vi "FEA_Model_Sample.vi"(8 "error in (no error)":errorcluster, 9 "include extremes":bool=TRUE, 10 "standard_deviation":dbl, 11 "FEA_Model in":refnum<class "FEA_Model.lvclass">) -> (0 "error out":errorcluster, 3 "FEA_Model out":refnum<class "FEA_Model.lvclass">)   [LabVIEW 2021, in "FEA_Model.lvclass"]
uses:
  FEA_Model.lvclass
  FEA_Model.lvclass/FEA_Model.ctl
  de957b9d-3b39-418b-bf55-63c688e4ea67.vi
  fbdf095a-6d06-4ca0-9642-1e4932d1de12.vi
  <vilib>/gmath/statdist.llb/Normal PDF.vi
  <vilib>/Comparison/Less/Less Functor/Less Functor.lvclass
  <vilib>/gmath/NI_Gmath.lvlib
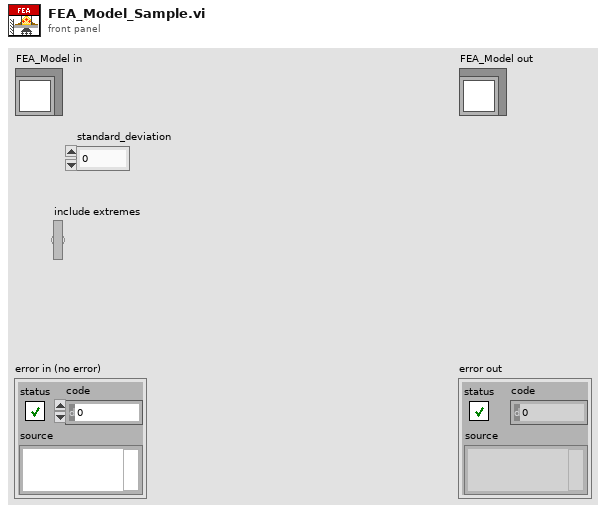
[diagram p1: front panel]
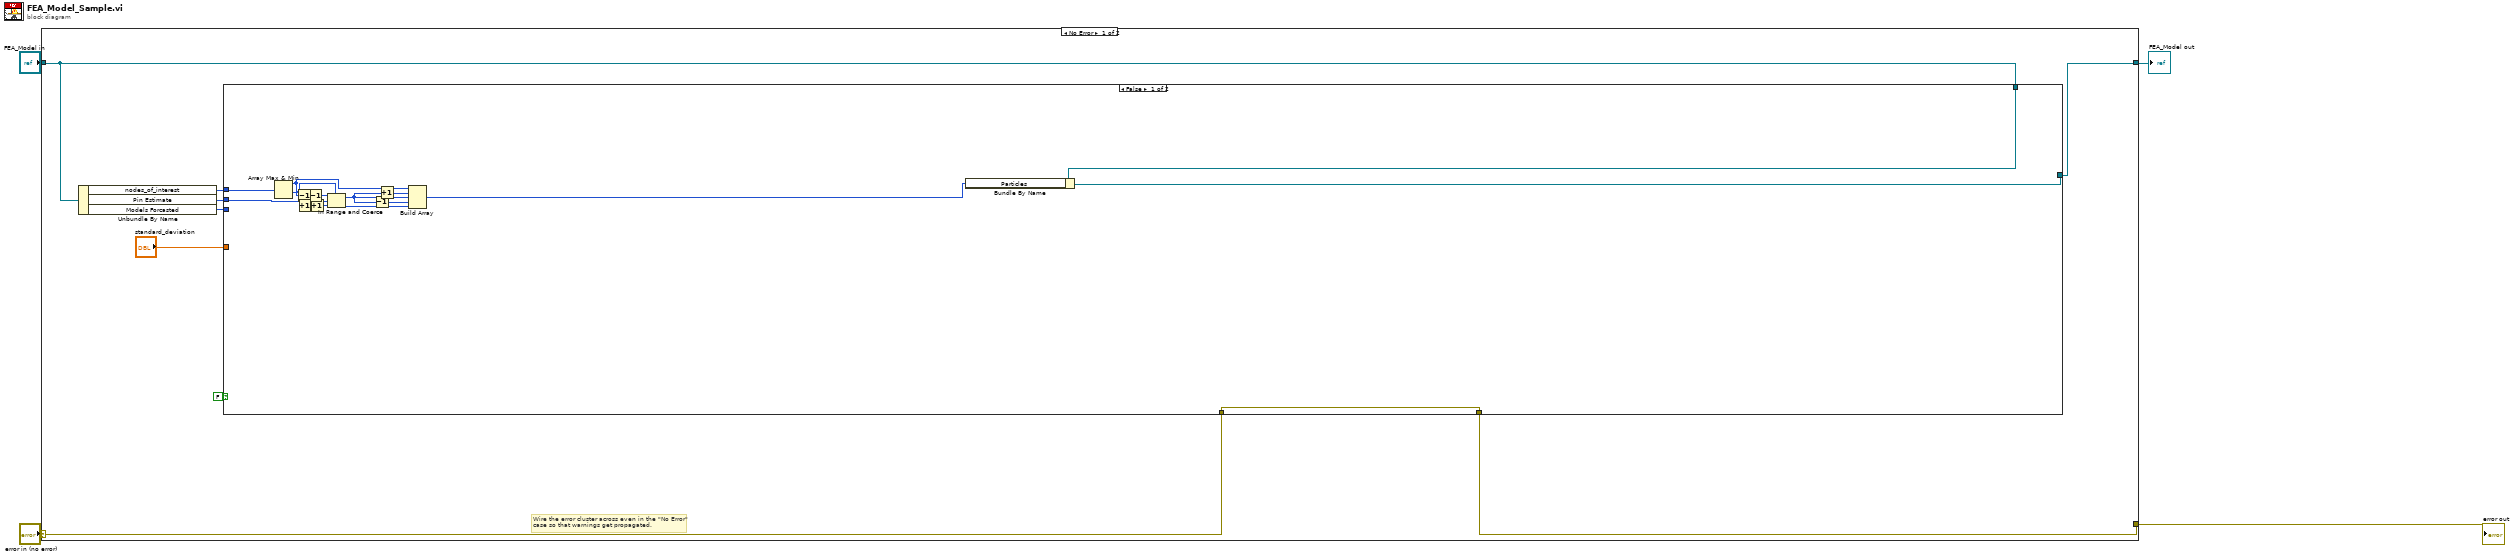
[diagram p0: block diagram]
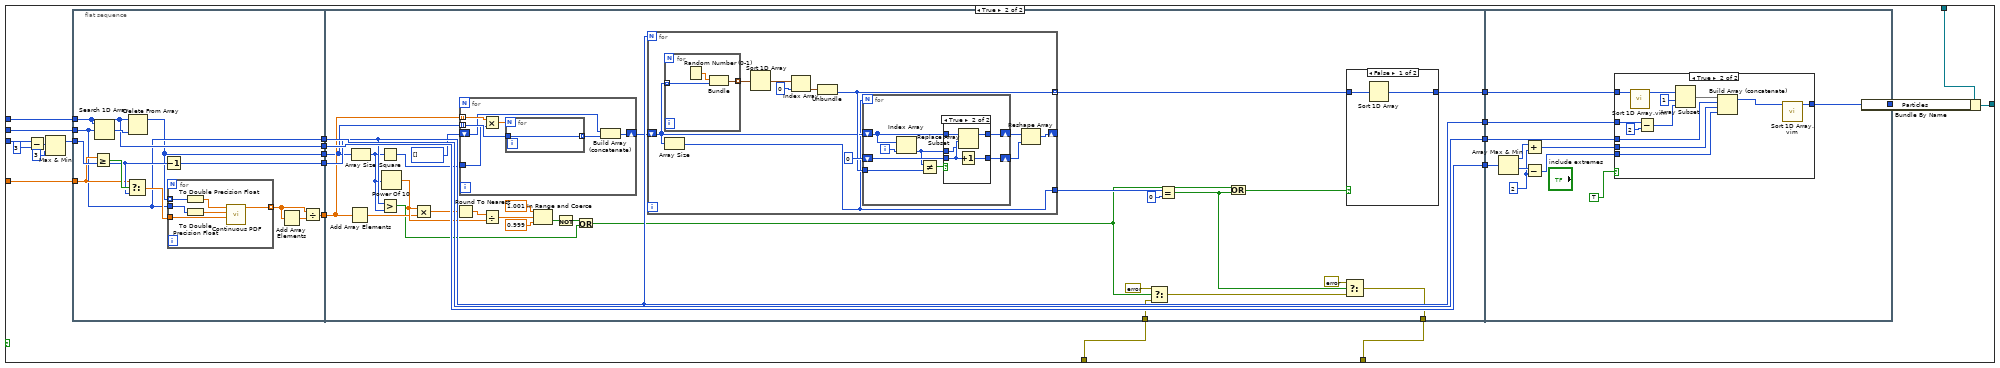
[diagram p2: hidden frame]
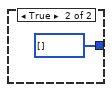
[diagram p3: hidden frame]
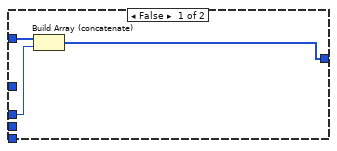
[diagram p5: hidden frame]
diagram:
  n1 = case shown="No Error" "error in (no error)" {
    selector: "error in (no error)" -> [w9 w167]
    tunnel: [w8 w167] -> w3
    tunnel: [w5 w166] -> w1
    tunnel: "FEA_Model in" -> [w6 w166]
    frame No Error {
      # "Wire the error cluster across even in the \"No Error\"\ncase so that warnings get propagated."
      n2 = Unbundle By Name(w6) -> ("nodes_of_interest"=w13:i32[], "Pin Estimate"=w12:i32, "Models Forcasted"=w10:i32)
      n3 = case shown="False" FALSE {
        tunnel: w13 -> [w28 w41]
        tunnel: w12 -> [w24 w40]
        tunnel: "standard_deviation" -> [_ w39]
        tunnel: [w27 w34] -> w5
        tunnel: w10 -> [_ w33]
        tunnel: w9 -> [w25 w37]
        tunnel: [w25 w36] -> w8
        tunnel: w6 -> [w26 w35]
        frame False {
          n4 = Array Max & Min(array=w28) -> (max value=w22:i32, min value=w21:i32)  [unwired: 2 out]
          n5 = Decrement(x=w22) -> (x-1=w19:i32)
          n6 = Increment(x=w21) -> (x+1=w20:i32)
          n7 = Decrement(x=w19) -> (x-1=w18:i32)
          n8 = Increment(x=w20) -> (x+1=w17:i32)
          n9 = In Range and Coerce(upper limit=w18, x=w24, lower limit=w17) -> (coerced(x)=w16:i32)  [unwired: 1 out]
          n10 = Decrement(x=w16) -> (x-1=w14:i32)
          n11 = Increment(x=w16) -> (x+1=w15:i32)
          n12 = Build Array(w22, w15, w16, w14, w21) -> (w23:i32[])
          n13 = Bundle By Name(cluster=w26, "Particles"=w23) -> (w27:refnum<class "FEA_Model.lvclass">)
        }
        frame True {
          n14 = Subtract(x=w33, y=3) -> (x-y=w32:i32)
          n15 = Max & Min(x=w32, y=3) -> (max(x,y)=w29:i32)  [unwired: 1 out]
          n16 = flat-sequence {
            tunnel: w41 -> [w57]
            tunnel: w40 -> [w54]
            tunnel: [w54] -> w50
            tunnel: [w53] -> w49
            tunnel: [w57] -> w48
            tunnel: [w51] -> w47
            tunnel: [w52] -> w46
            tunnel: w29 -> [w56]
            tunnel: w39 -> [w55]
            tunnel: [w96] -> w45
            tunnel: [w99] -> w44
            tunnel: [w97] -> w43
            tunnel: [w98] -> w42
            tunnel: w50 -> [w99]
            tunnel: w49 -> [w97]
            tunnel: w48 -> [w98]
            tunnel: w47 -> [w95]
            tunnel: w46 -> [w94]
            tunnel: [w70] -> w36
            tunnel: w37 -> [w69]
            tunnel: w45 -> [w150]
            tunnel: w44 -> [w149]
            tunnel: w43 -> [w148]
            tunnel: w42 -> [w147]
            tunnel: [w141] -> w38
            frame #0 {
              n17 = Greater Or Equal?(x=w55, y=w56) -> (x >= y?=w60:bool)
              n18 = Search 1D Array(1D array=w57, element=w54) -> (index of element=w62:i32)  [unwired: 1 in]
              n19 = Select(t=w55, s=w60, f=w56) -> (s? t:f=w61:dbl)
              n20 = Delete From Array(array=w57, index=w62) -> (array with subset deleted=w52:i32[])  [unwired: 1 in, 1 out]
              n21 = Decrement(x=w56) -> (x-1=w53:i32)
              n22 = for {
                tunnel: w52 -> [w65] mode=indexing
                tunnel: [w68] -> w59 mode=indexing
                tunnel: w54 -> [w64]
                tunnel: w61 -> [w67]
                n23 = To Double Precision Float(number=w65) -> (double precision float=w66:dbl)
                n24 = To Double Precision Float(number=w64) -> (double precision float=w63:dbl)
                n25 = call-poly <vilib>:"Continuous PDF.vi"("std"=w67, "mean"=w63, "x"=w66) -> ("pdf(x)"=w68:dbl)  [unwired: 7 in, 1 out]
              }
              n26 = Add Array Elements(numeric array=w59) -> (sum=w58:dbl)
              n27 = Divide(x=w59, y=w58) -> (x/y=w51:dbl[])
            }
            frame #1 {
              n28 = Add Array Elements(numeric array=w95) -> (sum=w84:dbl)
              n29 = Array Size(array=w94) -> (size(s)=w82:i32)
              n30 = Square(x=w82) -> (x^2=w83:i32)
              n31 = Greater?(x=w97, y=w82) -> (0:w81:bool)
              n32 = Power Of 10(x=w82) -> (10^x=w85:dbl)
              n33 = Multiply(x=w85, y=w84) -> (x*y=w87:dbl)
              n34 = Round To Nearest(number=w87) -> (nearest integer value=w86:dbl)
              n35 = for {
                tunnel: w95 -> [w138] mode=indexing
                tunnel: w94 -> [w136] mode=indexing
                shift-right: [w134] -> w79
                shift-left: i32[] [] -> [w133]
                tunnel: w83 -> [w132]
                n36 = Multiply(x=w138, y=w132) -> (x*y=w137:dbl)
                n37 = for {
                  N: w137 -> [_]
                  tunnel: w136 -> [w139]
                  tunnel: [w139] -> w135 mode=indexing
                }
                n38 = Build Array (concatenate)(w133, w135) -> (w134:i32[])
              }
              n39 = Divide(x=w86, y=w85) -> (x/y=w89:dbl)
              n40 = In Range and Coerce(upper limit=1.001, x=w89, lower limit=0.999) -> (In Range?=w92:bool)  [unwired: 1 out]
              n41 = Not(x=w92) -> (.not. x?=w93:bool)
              n42 = Or(x=w93, y=w81) -> (x .or. y?=w71:bool)
              n43 = for {
                N: w97 -> [_]
                tunnel: [w106] -> w74 mode=indexing
                shift-right: [w105] -> _
                shift-left: w79 -> [w104]
                tunnel: [w103] -> w76
                n44 = for {
                  tunnel: [w131] -> w113 mode=indexing
                  tunnel: w104 -> [w129] mode=indexing
                  n45 = Random Number (0-1)() -> (number: 0 to 1=w130:dbl)
                  n46 = Bundle("number: 0 to 1"=w130, w129) -> (w131:cluster{"number: 0 to 1":dbl, i32})  [unwired: 1 out]
                }
                n47 = Array Size(array=w104) -> (size(s)=w103:i32)
                n48 = Sort 1D Array(array=w113) -> (sorted array=w112:cluster{"number: 0 to 1":dbl, i32}[])
                n49 = Index Array(array=w112, index=0) -> (element=w111:cluster{"number: 0 to 1":dbl, i32})
                n50 = Unbundle(w111) -> (w106:i32)  [unwired: 1 out]
                n51 = for {
                  N: w103 -> [_]
                  shift-right: [w121] -> w108
                  shift-left: w104 -> [w119]
                  shift-right: [w117] -> w107
                  shift-left: 0 -> [w118]
                  tunnel: w106 -> [w116]
                  i -> [w120]
                  n52 = Index Array(array=w119, index=w120) -> (element=w114:i32)
                  n53 = Not Equal?(x=w114, y=w116) -> (x != y?=w115:bool)
                  n54 = case shown="True" w115 {
                    tunnel: w119 -> [w123 w128]
                    tunnel: [w123 w127] -> w121
                    tunnel: w118 -> [w122 w126]
                    tunnel: [w122 w125] -> w117
                    tunnel: w114 -> [_ w124]
                    frame False {
                    }
                    frame True {
                      n55 = Increment(x=w126) -> (x+1=w125:i32)
                      n56 = Replace Array Subset(array=w128, new element=w124, index=w126) -> (w127:i32[])
                    }
                  }
                }
                n57 = Reshape Array(w108, w107) -> (w105:i32[])
              }
              n58 = Select(t=errorcluster {"status"=FALSE, "code"=0, "source"="probability not equal to 1"} ("error constant"), s=w71, f=w69) -> (s? t:f=w75:errorcluster)
              n59 = Equal?(x=w76, y=0) -> (x = y?=w73:bool)
              n60 = Or(x=w71, y=w73) -> (x .or. y?=w72:bool)
              n61 = Select(t=errorcluster {"status"=FALSE, "code"=0, "source"="sampled more values than unique numbers"} ("error constant"), s=w73, f=w75) -> (s? t:f=w70:errorcluster)
              n62 = case shown="False" w72 {
                tunnel: [w100 i32[] []] -> w96
                tunnel: w74 -> [w101 _]
                frame False {
                  n63 = Sort 1D Array(array=w101) -> (sorted array=w100:i32[])
                }
                frame True {
                }
              }
            }
            frame #2 {
              w142 = 2 ("y")
              n64 = Array Max & Min(array=w147) -> (max value=w145:i32, min value=w146:i32)  [unwired: 2 out]
              n65 = Add(x=w145, y=w142) -> (x+y=w144:i32)
              n66 = Subtract(x=w146, y=w142) -> (x-y=w143:i32)
              n67 = case shown="True" TRUE ("include extremes") {
                tunnel: w150 -> [w153 w165]
                tunnel: [w151 w157] -> w141
                tunnel: w149 -> [w152 w158]
                tunnel: w144 -> [_ w155]
                tunnel: w143 -> [_ w154]
                tunnel: w148 -> [_ w162]
                frame False {
                  n68 = Build Array (concatenate)(w153, w152) -> (w151:i32[])
                }
                frame True {
                  n69 = call "Sort 1D Array.vim"("unsorted array"=w165) -> ("sorted array"=w164:i32[])  [unwired: 10 in]
                  n70 = Subtract(x=w162, y=2) -> (x-y=w161:i32)
                  n71 = Array Subset(array=w164, index=1, length=w161) -> (w159:i32[])
                  n72 = Build Array (concatenate)(w159, w158, w155, w154) -> (w156:i32[])
                  n73 = call "Sort 1D Array.vim"("unsorted array"=w156) -> ("sorted array"=w157:i32[])  [unwired: 10 in]
                }
              }
            }
          }
          n74 = Bundle By Name(cluster=w35, "Particles"=w38) -> (w34:refnum<class "FEA_Model.lvclass">)
        }
      }
    }
    frame Error {
    }
  }
  "error out" <- w3
  "FEA_Model out" <- w1
